vi "Sort 1D Array.vi"(7 "JSON Value in":refnum<class "JSON Value.lvclass">, 11 "error in (no error)":errorcluster) -> (8 "JSON Value out":refnum<class "JSON Value.lvclass">, 15 "error out":errorcluster)   [LabVIEW 2016, in "JSON Value.lvclass"]
doc: "Returns a sorted version of array with the elements arranged in ascending order. If array is an array of clusters, the function sorts the elements by comparing the first elements. If the first elements match, the function compares the second and subsequent elements."
uses:
  JSON Value.lvclass
  JSON Value.lvclass/JSON Value.ctl
  New JSON Value/New JSON String.vi
  Read Value/Read value as String.vi
  New JSON Value/New JSON Boolean.vi
  Read Value/Read value (Boolean).vi
  New JSON Value/New JSON Numeric.vi
  Read Value/Read value (Numeric).vi
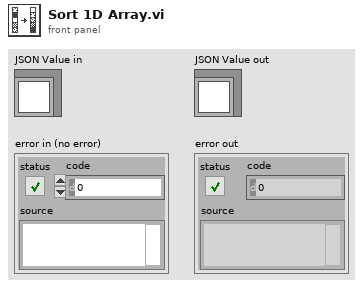
[diagram p1: front panel]
types:
  T1 = typedef "JSON Value.lvclass/JSON Types.ctl" = enum16{"String", "Numeric", "Boolean", "NULL", "Object", "Array"}
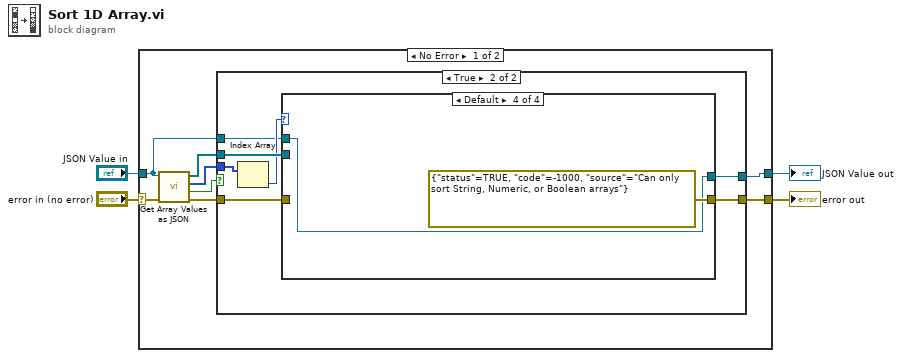
[diagram p0: block diagram]
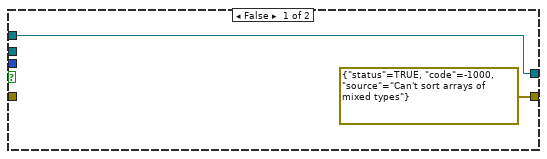
[diagram p2: hidden frame]
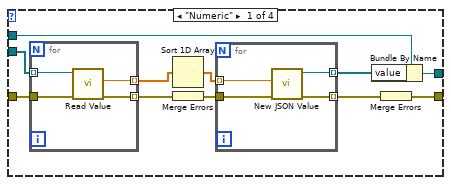
[diagram p3: hidden frame]
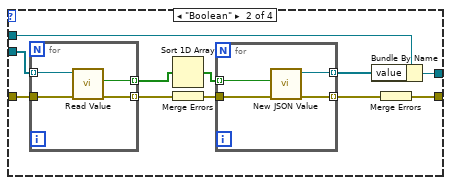
[diagram p4: hidden frame]
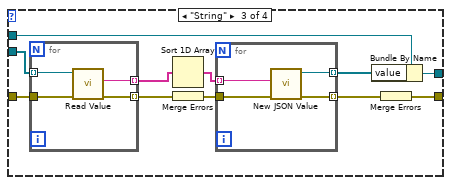
[diagram p5: hidden frame]
diagram:
  n1 = case shown="No Error" "error in (no error)" {
    selector: "error in (no error)" -> [w8 w82]
    tunnel: "JSON Value in" -> [w5 w81]
    tunnel: [w12 w81] -> w1
    tunnel: [w11 w82] -> w2
    frame No Error {
      n2 = call "Get Array Values as JSON.vi"("error in (no error)"=w8, "JSON Value in"=w5) -> ("error out"=w7:errorcluster, "single type?"=w9:bool, "types"=w10:T1[], "values"=w6:refnum<class "JSON Value.lvclass">[])  [unwired: 6 in]
      n3 = case shown="True" w9 {
        tunnel: w6 -> [_ w21]
        tunnel: [w13 w20] -> w12
        tunnel: w7 -> [_ w19]
        tunnel: [errorcluster {"status"=TRUE, "code"=-1000, "source"="Can't sort arrays of mixed types"} ("error IO") w18] -> w11
        tunnel: w10 -> [_ w17]
        tunnel: w5 -> [w13 w15]
        frame False {
        }
        frame True {
          n4 = Index Array(array=w17) -> (element=w16:T1)  [unwired: 1 in]
          n5 = case shown="Default" w16 {
            tunnel: w21 -> [w23 w42 w60 _]
            tunnel: [w30 w49 w70 w79] -> w20
            tunnel: w19 -> [w32 w51 w69 _]
            tunnel: [w31 w50 w68 errorcluster {"status"=TRUE, "code"=-1000, "source"="Can only sort String, Numeric, or Boolean arrays"} ("error IO")] -> w18
            tunnel: w15 -> [w22 w41 w61 w79]
            frame "Numeric" {
              n6 = for {
                tunnel: w23 -> [w37] mode=indexing
                tunnel: [w40] -> w29 mode=indexing
                tunnel: w32 -> [w39]
                tunnel: [w38] -> w27 mode=indexing
                n7 = call-poly "Read Value.vi"("error in (no error)"=w39, "JSON Numeric in"=w37) -> ("error out"=w38:errorcluster, "value"=w40:dbl)  [unwired: 8 in]
              }
              n8 = Sort 1D Array(array=w29) -> (sorted array=w28:dbl[])
              n9 = Merge Errors(w27) -> (w26:errorcluster)
              n10 = for {
                tunnel: w28 -> [w36] mode=indexing
                tunnel: [w35] -> w24 mode=indexing
                tunnel: w26 -> [w34]
                tunnel: [w33] -> w25 mode=indexing
                n11 = call-poly "New JSON Value.vi"("error in (no error)"=w34, "value"=w36) -> ("error out"=w33:errorcluster, "JSON Value out"=w35:refnum<class "JSON Value.lvclass">)  [unwired: 8 in]
              }
              n12 = Bundle By Name(cluster=w22, "value"=w24) -> (w30:refnum<class "JSON Value.lvclass">)
              n13 = Merge Errors(w25) -> (w31:errorcluster)
            }
            frame "Boolean" {
              n14 = for {
                tunnel: w42 -> [w56] mode=indexing
                tunnel: [w59] -> w48 mode=indexing
                tunnel: w51 -> [w58]
                tunnel: [w57] -> w46 mode=indexing
                n15 = call-poly "Read Value.vi"("error in (no error)"=w58, "JSON Boolean in"=w56) -> ("error out"=w57:errorcluster, "value"=w59:bool)  [unwired: 8 in]
              }
              n16 = Sort 1D Array(array=w48) -> (sorted array=w47:bool[])
              n17 = Merge Errors(w46) -> (w45:errorcluster)
              n18 = for {
                tunnel: w47 -> [w55] mode=indexing
                tunnel: [w54] -> w43 mode=indexing
                tunnel: w45 -> [w53]
                tunnel: [w52] -> w44 mode=indexing
                n19 = call-poly "New JSON Value.vi"("error in (no error)"=w53, "value"=w55) -> ("error out"=w52:errorcluster, "JSON Value out"=w54:refnum<class "JSON Value.lvclass">)  [unwired: 8 in]
              }
              n20 = Bundle By Name(cluster=w41, "value"=w43) -> (w49:refnum<class "JSON Value.lvclass">)
              n21 = Merge Errors(w44) -> (w50:errorcluster)
            }
            frame "String" {
              n22 = for {
                tunnel: w60 -> [w75] mode=indexing
                tunnel: [w78] -> w67 mode=indexing
                tunnel: w69 -> [w77]
                tunnel: [w76] -> w65 mode=indexing
                n23 = call-poly "Read Value.vi"("error in (no error)"=w77, "JSON String in"=w75) -> ("error out"=w76:errorcluster, "value"=w78:string)  [unwired: 8 in]
              }
              n24 = Sort 1D Array(array=w67) -> (sorted array=w66:string[])
              n25 = Merge Errors(w65) -> (w64:errorcluster)
              n26 = for {
                tunnel: w66 -> [w74] mode=indexing
                tunnel: [w73] -> w62 mode=indexing
                tunnel: w64 -> [w72]
                tunnel: [w71] -> w63 mode=indexing
                n27 = call-poly "New JSON Value.vi"("error in (no error)"=w72, "value"=w74) -> ("error out"=w71:errorcluster, "JSON Value out"=w73:refnum<class "JSON Value.lvclass">)  [unwired: 8 in]
              }
              n28 = Bundle By Name(cluster=w61, "value"=w62) -> (w70:refnum<class "JSON Value.lvclass">)
              n29 = Merge Errors(w63) -> (w68:errorcluster)
            }
            frame Default {
            }
          }
        }
      }
    }
    frame Error {
    }
  }
  "error out" <- w2
  "JSON Value out" <- w1
